vi "CableEnd.vi"(11 "Raw":dbl[](array[numeric])) -> (1 "CableEnd":dbl, 2 "Filtered":dbl[](array[numeric]), 3 "CableEndSet":bool)   [LabVIEW 2011]
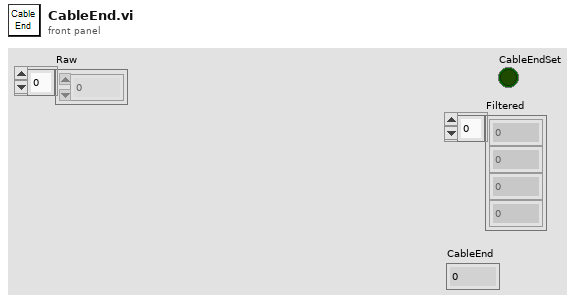
[diagram p1: front panel]
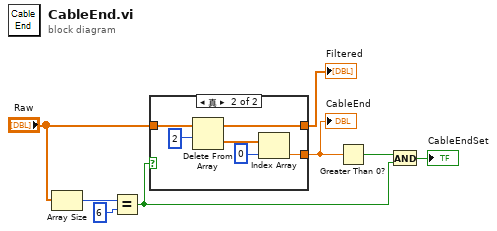
[diagram p0: block diagram]
diagram:
  n1 = Array Size(array="Raw") -> (size(s)=w8:i32)
  n2 = Equal?(x=w8, y=6) -> (x = y?=w1:bool)
  n3 = case shown="真" w1 {
    tunnel: "Raw" -> [w9 w15]
    tunnel: [w9 w13] -> w6
    tunnel: [_ w10] -> w4
    frame False {
    }
    frame True {
      n4 = Delete From Array(array=w15, length=2 ("长度")) -> (deleted portion=w12:dbl[], array with subset deleted=w13:dbl[])  [unwired: 1 in]
      n5 = Index Array(array=w12, index=0 ("索引")) -> (element=w10:dbl)
    }
  }
  "CableEnd" <- w4
  "Filtered" <- w6
  n6 = Greater Than 0?(x=w4) -> (x > 0?=w3:bool)
  n7 = And(x=w3, y=w1) -> (x .and. y?=→"CableEndSet":bool)
